vi "DrawPiePlot.vi"(0 "reference in":refnum<class "LcWebView.lvclass">, 1 "PiePlot.PlotLabels":string[](array[string]), 2 "PiePlot.Dataset":dbl[][](array[numeric]), 3 "PiePlot.DatasetLabels":string[](array[string]), 5 "Error In":errorcluster, 6 "GenericPlotOptions":T1, 7 "PiePlot.PlotColours":u32[](array[numeric]), 8 "PiePlotOptions":T3) -> (14 "reference out":refnum<class "LcWebView.lvclass">, 19 "Error Out":errorcluster)   [LabVIEW 2019, in "LcWebView.lvclass"]
uses:
  LcWebView.lvclass
  Program Files/National Instruments/LabVIEW 2020/user.lib/_LabVIEWCommon/LcHTMLPlot/HTMLPlot_class/Controls/LegendPosition.ctl
  Program Files/National Instruments/LabVIEW 2020/user.lib/_LabVIEWCommon/LcHTMLPlot/HTMLPlot_class/HTMLPlot.lvclass
  Program Files/National Instruments/LabVIEW 2020/user.lib/_LabVIEWCommon/LcHTMLPlot/HTMLPlot_class/Controls/GenericPlotOptions.ctl
  Program Files/National Instruments/LabVIEW 2020/user.lib/_LabVIEWCommon/LcHTMLPlot/HTMLPlot_class/Controls/PiePlotOptions.ctl
  c4f0e229-e96c-4f69-afb9-f3a8197e14da.vi
  ctrls/PiePlotOption.ctl
  ctrls/GenericPlotOption.ctl
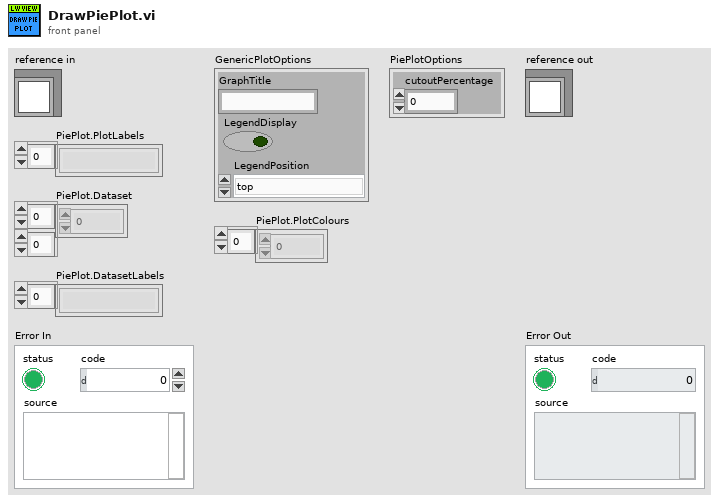
[diagram p1: front panel]
types:
  T1 = typedef "LcWebView.lvclass/GenericPlotOption.ctl" = cluster{"GraphTitle":string, "LegendDisplay":bool, "LegendPosition":T2}
  T2 = typedef "HTMLPlot.lvclass/LegendPosition.ctl" = enum16{"top", "right", "left", "bottom"}
  T3 = typedef "LcWebView.lvclass/PiePlotOption.ctl" = cluster{"cutoutPercentage":i32}
  T4 = typedef "HTMLPlot.lvclass/GenericPlotOptions.ctl" = cluster{"GraphTitle":string, "LegendDisplay":bool, "LegendPosition":T2}
  T5 = typedef "HTMLPlot.lvclass/PiePlotOptions.ctl" = cluster{"cutoutPercentage":i32}
  T6 = cluster{"action":string, "PlotData":string, "GenericPlotOptions":T4, "PiePlotOptions":T5}
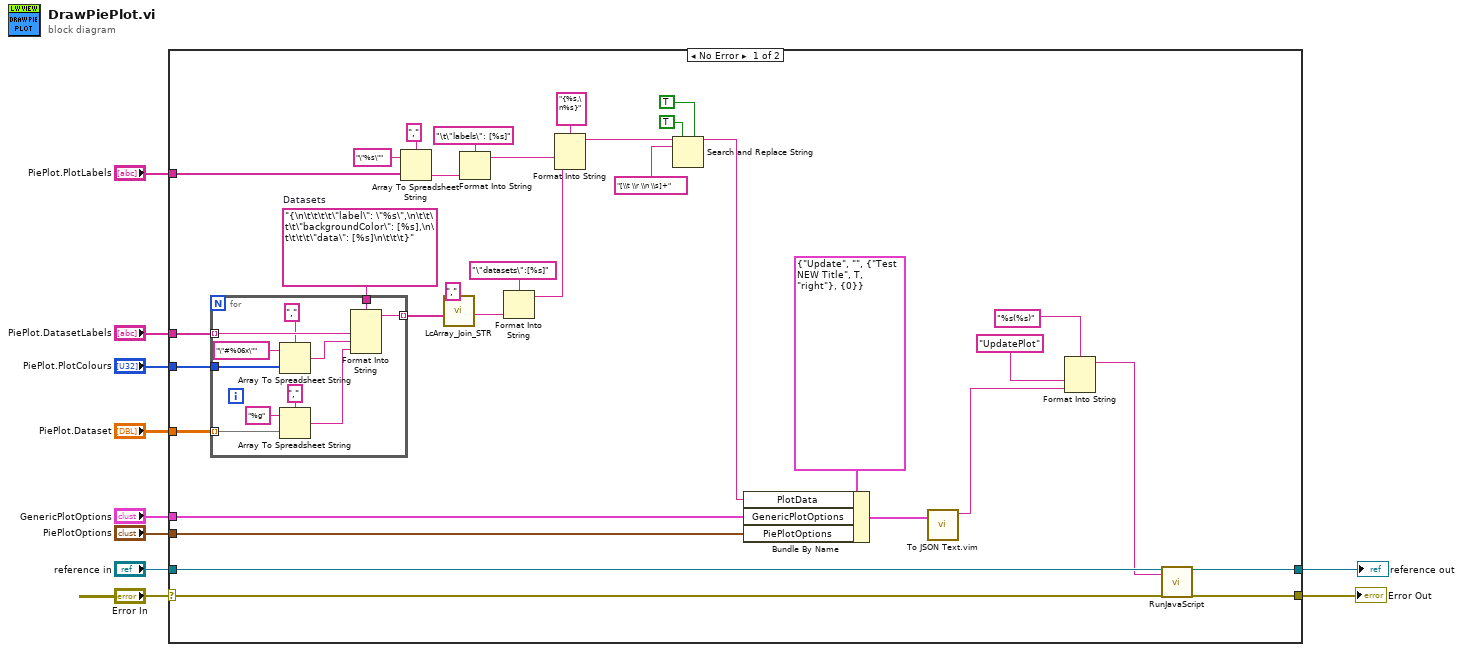
[diagram p0: block diagram]
diagram:
  n1 = case shown="No Error" "Error In" {
    selector: "Error In" -> [w19 w56]
    tunnel: [w12 w56] -> w4
    tunnel: [w13 w55] -> w1
    tunnel: "reference in" -> [w18 w55]
    tunnel: "PiePlot.Dataset" -> [w31 _]
    tunnel: "PiePlot.PlotColours" -> [w30 _]
    tunnel: "PiePlot.DatasetLabels" -> [w29 _]
    tunnel: "PiePlot.PlotLabels" -> [w28 _]
    tunnel: "GenericPlotOptions" -> [w22 _]
    tunnel: "PiePlotOptions" -> [w20 _]
    frame No Error {
      w32 = "{\n\t\t\t\t\"label\": \"%s\",\n\t\t\t\t\"backgroundColor\": [%s],\n\t\t\t\t\"data\": [%s]\n\t\t\t}"  # Datasets
      n2 = for {
        tunnel: w31 -> [w52] mode=indexing
        tunnel: w30 -> [w45]
        tunnel: w29 -> [w51] mode=indexing
        tunnel: [w49] -> w37 mode=indexing
        tunnel: w32 -> [w48]
        n3 = Array To Spreadsheet String(delimiter (Tab)=",", array=w45, 3:"\"#%06x\"" ("format string")) -> (spreadsheet string=w44:string)
        n4 = Array To Spreadsheet String(delimiter (Tab)=",", array=w52, 3:"%g" ("format string")) -> (spreadsheet string=w50:string)
        n5 = Format Into String(format string=w48, w51, w44, w50) -> (resulting string=w49:string)  [unwired: 2 in, 1 out]
      }
      n6 = Array To Spreadsheet String(delimiter (Tab)=",", array=w28, 3:"\"%s\"" ("format string")) -> (spreadsheet string=w39:string)
      n7 = call "LcArray_Join_STR.vi"("separator"=",", "Array"=w37) -> ("joined string"=w36:string)  [unwired: 8 in, 1 out]
      n8 = Format Into String(format string="\t\"labels\": [%s]", w39) -> (resulting string=w42:string)  [unwired: 2 in, 1 out]
      n9 = Format Into String(format string="\"datasets\":[%s]", w36) -> (resulting string=w34:string)  [unwired: 2 in, 1 out]
      n10 = Format Into String(format string="{%s,\n%s}", w42, w34) -> (resulting string=w21:string)  [unwired: 2 in, 1 out]
      n11 = Search and Replace String(replace all?=TRUE ("replace all? (F)"), multiline?=TRUE ("multiline? (F)"), input string=w21, search string="[\\t \\r \\n \\s]+") -> (result string=w27:string)  [unwired: 4 in, 3 out]
      n12 = Bundle By Name(cluster=T6 {"action"="Update", "PlotData"="", "GenericPlotOptions"={"GraphTitle"="Test NEW Title", "LegendDisplay"=TRUE, "LegendPosition"=enum."right"}, "PiePlotOptions"={"cutoutPercentage"=0}}, "PlotData"=w27, "GenericPlotOptions"=w22, "PiePlotOptions"=w20) -> (w17:T6)
      n13 = call "To JSON Text.vim"("Anything"=w17) -> ("<JSON>"=w14:string)  [unwired: 9 in, 1 out]
      n14 = Format Into String(format string="%s(%s)", "UpdatePlot" ("input 1"), w14) -> (resulting string=w11:string)  [unwired: 2 in, 1 out]
      n15 = call-dynamic "RunJavaScript.vi"("reference in"=w18, "Java Script Function"=w11, "Error In"=w19) -> ("reference out"=w13:refnum<class "LcWebView.lvclass">, "Error Out"=w12:errorcluster)  [unwired: 13 in, 2 out]
    }
    frame Error {
    }
  }
  "Error Out" <- w4
  "reference out" <- w1
